vi "UTILITY Convert String to Time.vi"(6 "date/time string":string, 8 "Error In":errorcluster) -> (0 "Error Out":errorcluster, 2 "Time Stamp Float":ext, 4 "Resulting Time Stamp":timestamp)   [LabVIEW 2016]
doc: "This VI convert a date/time string back to a time stamp."
uses:
  <vilib>/Utility/miscctls.llb/LVDateTimeRec.ctl
panel:
  # "This control should have data in the form:\n4/30/2004 7:48:47 PM"
  # "01/22/2018 13:08:07.052"
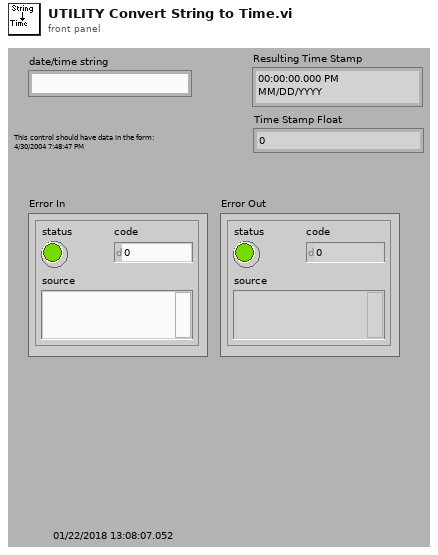
[diagram p1: front panel]
types:
  T1 = typedef "LVDateTimeRec.ctl" = cluster{"fractional second":dbl, "second":i32, "minute":i32, "hour":i32, "day of month":i32, "month":i32, "year":i32, "day of week":i32, "day of year":i32, "DST":i32}
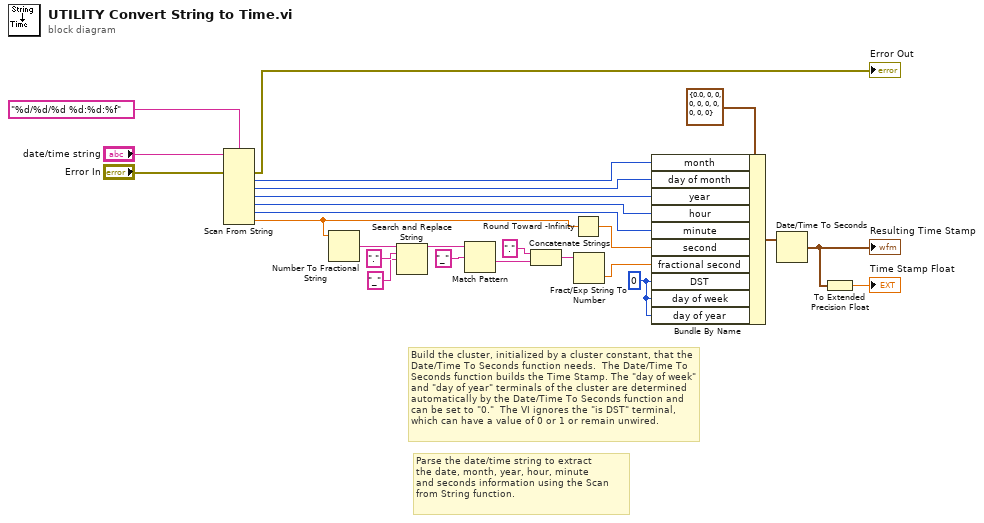
[diagram p0: block diagram]
diagram:
  w17 = 0
  # "Build the cluster, initialized by a cluster constant, that the Date/Time To Seconds function needs.  The Date/Time To Seconds function builds the Time Stamp. The \"day of week\" and \"day of year\" terminals of the cluster are determined automatically by the Date/Time To Seconds function and can be set to \"0.\"  The VI ignores the \"is DST\" terminal, which can have a value of 0 or 1 or remain unwired."
  # "Parse the date/time string to extract \nthe date, month, year, hour, minute \nand seconds information using the Scan\nfrom String function."
  n1 = Scan From String "Scan From String"(format string="%d/%d/%d %d:%d:%f", input string="date/time string", error in="Error In") -> (error out=→"Error Out":errorcluster, output 1=w23:i32, output 2=w22:i32, output 3=w21:i32, output 4=w20:i32, output 5=w19:i32, output 6=w14:dbl)  [unwired: 7 in, 2 out]
  n2 = Number To Fractional String(number=w14) -> (F-format string=w10:string)  [unwired: 3 in]
  n3 = Search and Replace String(input string=w10, search string=".", replace string="_" ("replace string (\"\")")) -> (result string=w7:string)  [unwired: 5 in, 3 out]
  n4 = Match Pattern(string=w7, regular expression="_") -> (after substring=w12:string)  [unwired: 1 in, 3 out]
  n5 = Concatenate Strings("." ("string"), w12) -> (w11:string)
  n6 = Round Toward -Infinity(1:w14) -> (0:w15:dbl)
  n7 = Fract/Exp String To Number(string=w11) -> (number=w5:dbl)  [unwired: 3 in, 1 out]
  n8 = Bundle By Name(cluster=T1 {"fractional second"=0.0, "second"=0, "minute"=0, "hour"=0, "day of month"=0, "month"=0, "year"=0, "day of week"=0, "day of year"=0, "DST"=0} ("date time rec"), "month"=w23, "day of month"=w22, "year"=w21, "hour"=w20, "minute"=w19, "second"=w15, "fractional second"=w5, "DST"=w17, "day of week"=w17, "day of year"=w17) -> (w16:T1)
  n9 = Date/Time To Seconds(2:w16) -> (0:w2:timestamp)  [unwired: 1 in]
  "Resulting Time Stamp" <- w2
  n10 = To Extended Precision Float(1:w2) -> (0:→"Time Stamp Float":ext)
